vi "Is Closed.vi"(11 "Enclave in":refnum<class "Enclave.lvclass">) -> (2 "Is Closed?":bool)   [LabVIEW 2022 SP3, in "Enclave.lvlib" / "Enclave.lvclass"]
uses:
  Enclave.lvclass
  Enclave.lvclass/Enclave.ctl
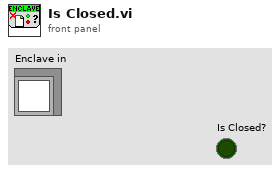
[diagram p1: front panel]
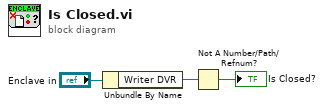
[diagram p0: block diagram]
diagram:
  n1 = Unbundle By Name("Enclave in") -> ("Writer DVR"=w2:refnum<data-value>)
  n2 = Not A Number/Path/Refnum?(number/path/refnum=w2) -> (NaN/Path/Refnum?=→"Is Closed?":bool)
